vi "PositionControlRelative.vi"(7 "Mode":T1=enum."Read Pos", 8 "error in (no error)":errorcluster, 9 "Calibration":cluster{dbl, "MicrostepMode":u32}[](array[cluster]), 10 "Move to":sgl[](array[numeric]), 11 "IDs":i32[](array[numeric])) -> (0 "error out":errorcluster, 2 "Position":sgl[](array[numeric]), 3 "Success?":bool)   [LabVIEW 2020]
uses:
  PosCtrlOptions.ctl
  libximc.lvlib
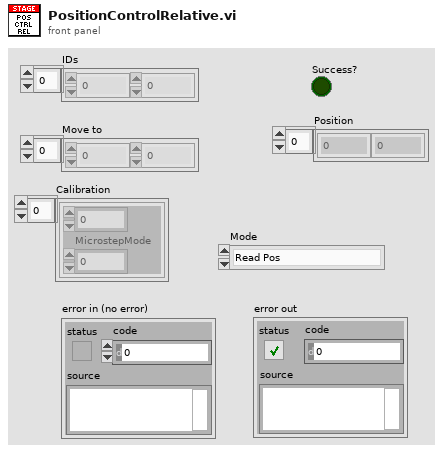
[diagram p1: front panel]
types:
  T1 = typedef "PosCtrlOptions.ctl" = enum16{"Move X", "Move Y", "Both X and Y", "Read Pos", "None"}
  T2 = cluster{"MoveSts":u32, "MvCmdSts":u32, "PWRSts":u32, "EncSts":u32, "WindSts":u32, "CurPosition":sgl, "EncPosition":i64, "CurSpeed":sgl, "Ipwr":i32, "Upwr":i32, "Iusb":i32, "Uusb":i32, "CurT":i32, "Flags":u32, "GPIOFlags":u32, "CmdBufFreeSpace":u32}
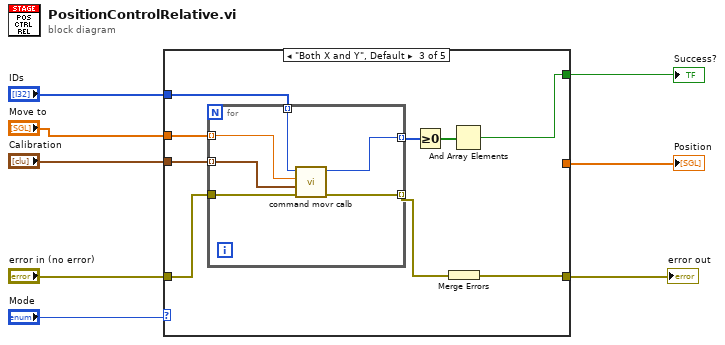
[diagram p0: block diagram]
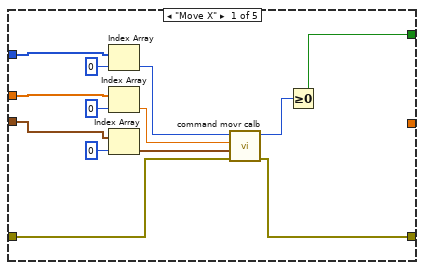
[diagram p2: hidden frame]
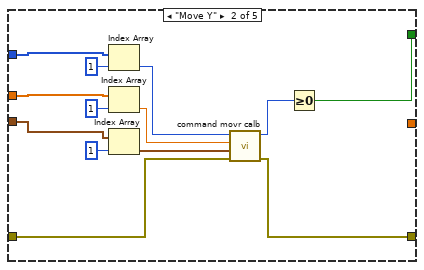
[diagram p3: hidden frame]
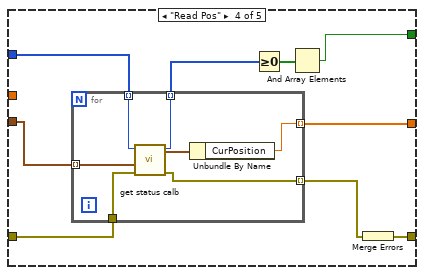
[diagram p4: hidden frame]
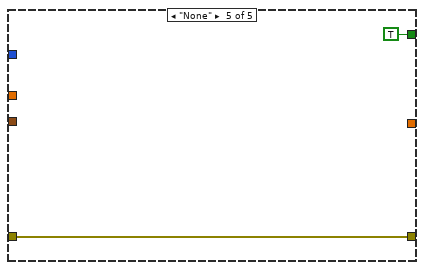
[diagram p5: hidden frame]
diagram:
  n1 = case shown="\"Both X and Y\", Default" "Mode" {
    tunnel: "Move to" -> [w17 w30 w43 _ _]
    tunnel: "IDs" -> [w21 w34 w42 w55 _]
    tunnel: "error in (no error)" -> [w12 w25 w41 w53 w67]
    tunnel: [w11 w24 w38 w52 w67] -> w3
    tunnel: "Calibration" -> [w14 w27 w39 w54 _]
    tunnel: [w9 w23 w35 w57 TRUE] -> w2
    tunnel: [_ _ _ w50 _] -> w1
    frame "Move X" {
      n2 = Index Array(array=w21, index=0) -> (element=w19:i32)
      n3 = Index Array(array=w17, index=0) -> (element=w16:sgl)
      n4 = Index Array(array=w14, index=0) -> (element=w13:cluster{dbl, "MicrostepMode":u32})
      n5 = call "command movr calb.vi"("error in (no error)"=w12, "calibration"=w13, "DeltaPosition"=w16, "id"=w19) -> ("error out"=w11:errorcluster, "function return"=w10:i32)  [unwired: 6 in]
      n6 = Greater Or Equal To 0?(x=w10) -> (x >= 0?=w9:bool)
    }
    frame "Move Y" {
      n7 = Index Array(array=w34, index=1) -> (element=w32:i32)
      n8 = Index Array(array=w30, index=1) -> (element=w29:sgl)
      n9 = Index Array(array=w27, index=1) -> (element=w26:cluster{dbl, "MicrostepMode":u32})
      n10 = call "command movr calb.vi"("error in (no error)"=w25, "calibration"=w26, "DeltaPosition"=w29, "id"=w32) -> ("error out"=w24:errorcluster, "function return"=w22:i32)  [unwired: 6 in]
      n11 = Greater Or Equal To 0?(x=w22) -> (x >= 0?=w23:bool)
    }
    frame "Both X and Y", Default {
      n12 = for {
        tunnel: w43 -> [w49] mode=indexing
        tunnel: [w48] -> w40 mode=indexing
        tunnel: w42 -> [w47] mode=indexing
        tunnel: w41 -> [w46]
        tunnel: [w45] -> w36 mode=indexing
        tunnel: w39 -> [w44] mode=indexing
        n13 = call "command movr calb.vi"("error in (no error)"=w46, "calibration"=w44, "DeltaPosition"=w49, "id"=w47) -> ("error out"=w48:errorcluster, "function return"=w45:i32)  [unwired: 6 in]
      }
      n14 = Greater Or Equal To 0?(x=w36) -> (x >= 0?=w37:bool[])
      n15 = Merge Errors(w40) -> (w38:errorcluster)
      n16 = And Array Elements(Boolean array=w37) -> (logical AND=w35:bool)
    }
    frame "Read Pos" {
      n17 = for {
        tunnel: w55 -> [w65] mode=indexing
        tunnel: [w64] -> w51 mode=indexing
        tunnel: w53 -> [w62]
        tunnel: w54 -> [w61] mode=indexing
        tunnel: [w60] -> w50 mode=indexing
        tunnel: [w59] -> w56 mode=indexing
        n18 = call "get status calb.vi"("error in (no error)"=w62, "calibration"=w61, "id"=w65) -> ("error out"=w64:errorcluster, "status out"=w63:T2, "function return"=w59:i32)  [unwired: 6 in]
        n19 = Unbundle By Name(w63) -> ("CurPosition"=w60:sgl)
      }
      n20 = Greater Or Equal To 0?(x=w56) -> (x >= 0?=w58:bool[])
      n21 = And Array Elements(Boolean array=w58) -> (logical AND=w57:bool)
      n22 = Merge Errors(w51) -> (w52:errorcluster)
    }
    frame "None" {
    }
  }
  "error out" <- w3
  "Success?" <- w2
  "Position" <- w1
